vi "_CSMObj-Clone Worker.vi"(8 "Error In":errorcluster caption="error in (no error)", 11 "CSMObj In":T1={"info"={"Module Name"="", "Requested Name"="", "Group Name"="", "Mode"=enum."Stand Alone", "Allowed Messages"=[]}, "Refs"={"WatchDogQ"=refnum, "CSMDataDVR"=refnum, "Queue"={"HPriorityQ"=refnum, "LowPriorityQ"=refnum}, "GroupDataDVR"=refnum, "TagMap"=refnum, "ExitEvent"=refnum, "NewStateEvent"=refnum, "StatusChangeEvent"=refnum}}) -> (0 "error out":errorcluster, 2 "Output Cluster":T1={"info"={"Module Name"="", "Requested Name"="", "Group Name"="", "Mode"=enum."Stand Alone", "Allowed Messages"=[]}, "Refs"={"WatchDogQ"=refnum, "CSMDataDVR"=refnum, "Queue"={"HPriorityQ"=refnum, "LowPriorityQ"=refnum}, "GroupDataDVR"=refnum, "TagMap"=refnum, "ExitEvent"=refnum, "NewStateEvent"=refnum, "StatusChangeEvent"=refnum}}, 3 "CSMObj Out":T1={"info"={"Module Name"="", "Requested Name"="", "Group Name"="", "Mode"=enum."Stand Alone", "Allowed Messages"=[]}, "Refs"={"WatchDogQ"=refnum, "CSMDataDVR"=refnum, "Queue"={"HPriorityQ"=refnum, "LowPriorityQ"=refnum}, "GroupDataDVR"=refnum, "TagMap"=refnum, "ExitEvent"=refnum, "NewStateEvent"=refnum, "StatusChangeEvent"=refnum}})   [LabVIEW 2017, in "Communicable State Machine.lvlib"]
uses:
  Communicable State Machine.lvlib
  _CSMObj.ctl
  _CSMObj-Info.ctl
  Typedef/_CSM_MODE.ctl
  _CSMObj-Refs.ctl
  _CSMObj-Data.ctl
  Priority Queue/Priority Queue.ctl
  Typedef/_Cross CSM State Data.ctl
  Typedef/_CSM_MSG_TYPE.ctl
  Typedef/_Cross CSM State Response.ctl
  Typedef/_CSM_Response Source Message.ctl
  Priority Queue/def-Data(LowPRI-Q).ctl
  _CSMObj-ModeData.ctl
  Typedef/_CSM Status Change Event Data.ctl
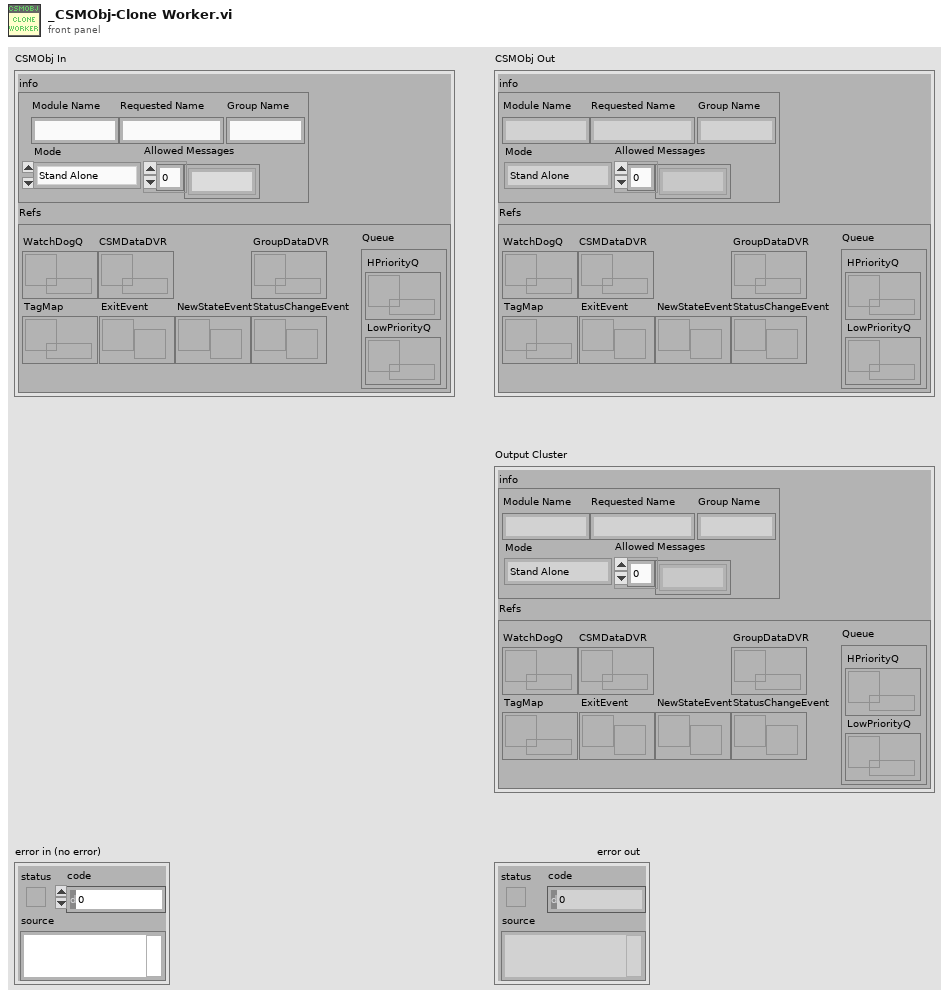
[diagram p1: front panel]
types:
  T1 = typedef "Communicable State Machine.lvlib/_CSMObj.ctl" = cluster{"info":T2, "Refs":T4}
  T2 = typedef "Communicable State Machine.lvlib/_CSMObj-Info.ctl" = cluster{"Module Name":string, "Requested Name":string, "Group Name":string, "Mode":T3, "Allowed Messages":string[]}
  T3 = typedef "Communicable State Machine.lvlib/_CSM_MODE.ctl" = enum16{"Not Exist", "Stand Alone", "CSM", "Worker", "Worker Agent", "Chain Node", "Chain"}
  T4 = typedef "Communicable State Machine.lvlib/_CSMObj-Refs.ctl" = cluster{"WatchDogQ":refnum<queue>, "CSMDataDVR":refnum<data-value>, "Queue":T5, "GroupDataDVR":refnum<data-value>, "TagMap":refnum<data-value>, "ExitEvent":refnum<user-event>, "NewStateEvent":refnum<user-event>, "StatusChangeEvent":refnum<user-event>}
  T5 = typedef "Communicable State Machine.lvlib/Priority Queue.ctl" = cluster{"HPriorityQ":refnum<queue>, "LowPriorityQ":refnum<queue>}
  T6 = typedef "Communicable State Machine.lvlib/_CSMObj-Data.ctl" = cluster{"RemoteMessge?":bool, "error":errorcluster, "Return State":string, "Initialized":enum16{"Initializing", "Ready", "Exiting"}}
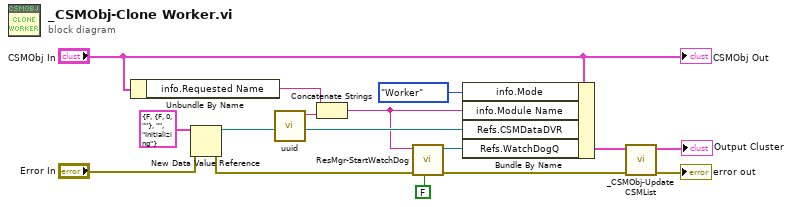
[diagram p0: block diagram]
diagram:
  n1 = Unbundle By Name("CSMObj In") -> ("info.Requested Name"=w7:string)
  n2 = New Data Value Reference(data value=T6 {"RemoteMessge?"=FALSE, "error"={"status"=FALSE, "code"=0, "source"=""}, "Return State"="", "Initialized"=enum."Initializing"} ("CSMObj-Data"), error in="Error In") -> (data value reference=w10:refnum<data-value>, error out=w11:errorcluster)
  n3 = call "uuid.vi"() -> ("UUID"=w15:string)  [unwired: 11 in]
  n4 = Concatenate Strings(w7, w15) -> (w9:string)
  n5 = call "ResMgr-StartWatchDog.vi"("Force?"=FALSE, "error in (no error)"=w11, "ModuleName"=w9) -> ("error out"=w5:errorcluster, "WatchDogQ"=w8:refnum<queue>)  [unwired: 7 in]
  n6 = Bundle By Name(cluster="CSMObj In", "info.Mode"=_CSM_MODE."Worker" ("Mode"), "info.Module Name"=w9, "Refs.CSMDataDVR"=w10, "Refs.WatchDogQ"=w8) -> (w3:T1)
  n7 = call "_CSMObj-Update CSMList.vi"("Error In"=w5, "CSMObj In"=w3) -> ("error out"=→"error out":errorcluster, "CSMObj Out"=→"Output Cluster":T1)  [unwired: 8 in]
  "CSMObj Out" <- "CSMObj In"
